vi "updateEndEventTime.vi"(8 "error in (no error)":errorcluster, 11 "RampAction in":refnum<class "RampAction.lvclass">) -> (0 "error out":errorcluster, 3 "RampAction out":refnum<class "RampAction.lvclass">)   [LabVIEW 2011, in "Views.lvlib" / "ScriptEditor.lvlib" / "RampAction.lvclass"]
uses:
  RampAction.lvclass
  Tools/Scripting/ScriptingEvent/ScriptEvents/Ramp/RampEvent/RampEvent.lvclass
  ActionPanel.lvclass
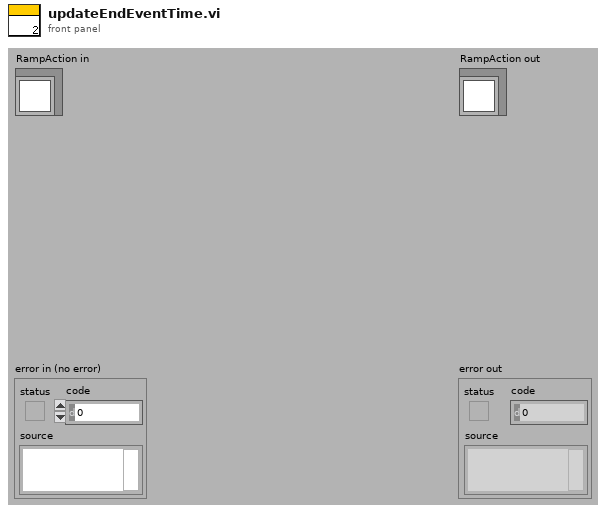
[diagram p1: front panel]
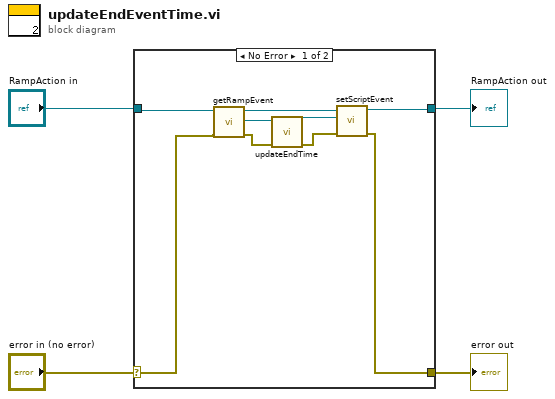
[diagram p0: block diagram]
diagram:
  n1 = case shown="No Error" "error in (no error)" {
    selector: "error in (no error)" -> [w7 w15]
    tunnel: [w6 w15] -> w3
    tunnel: [w5 w14] -> w1
    tunnel: "RampAction in" -> [w13 w14]
    frame No Error {
      n2 = call "getRampEvent.vi"("error in (no error)"=w7, "RampAction in"=w13) -> ("error out"=w11:errorcluster, "RampEvent"=w12:refnum<class "RampEvent.lvclass">, "RampAction out"=w10:refnum<class "RampAction.lvclass">)  [unwired: 7 in]
      n3 = call-dynamic "updateEndTime.vi"("error in (no error)"=w11, "RampEvent in"=w12) -> ("error out"=w8:errorcluster, "RampEvent out"=w9:refnum<class "RampEvent.lvclass">)  [unwired: 8 in]
      n4 = call "setScriptEvent.vi"("error in (no error)"=w8, "ScriptEvent.lvclass"=w9, "ActionPanel.lvclass in"=w10) -> ("error out"=w6:errorcluster, "ActionPanel.lvclass out"=w5:refnum<class "RampAction.lvclass">)  [unwired: 7 in]
    }
    frame Error {
    }
  }
  "error out" <- w3
  "RampAction out" <- w1
